vi "BRig_dataLC_ENL_PostR_OnOff_l1.vi"() -> (2 "output_ENL_PostR_OnOff":i32)   [LabVIEW 2014]
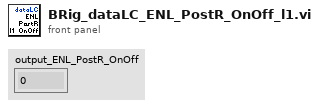
[diagram p1: front panel]
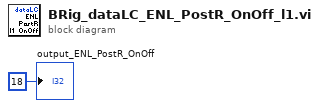
[diagram p0: block diagram]
diagram:
  "output_ENL_PostR_OnOff" <- 18 ("output_iBlock")
